vi "states FG.vi"(6 "exit in":bool, 8 "state # in":i32, 9 "subState in":T1, 10 "menu (get)":enum16{"set", "get"}(ring)=enum."get", 11 "Loop ID":i32) -> (0 "first call?":bool, 1 "exit out":bool, 2 "state # out":i32, 3 "subState out":T1=enum."driver control")   [LabVIEW 2013]
uses:
  typedefs/State Machine/subStates.ctl
panel:
  # "The All-Powerful Functional Global with all the States"
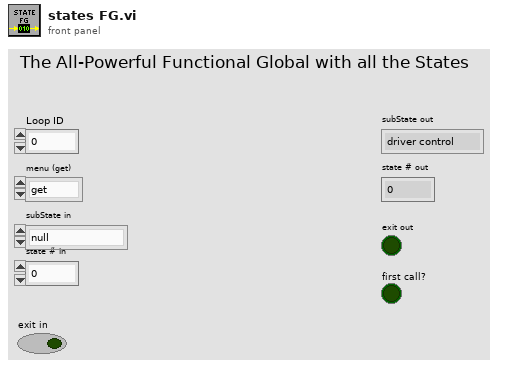
[diagram p1: front panel]
types:
  T1 = typedef "subStates.ctl" = enum16{"null", "wait", "driver control", "auto", "manual override", "hold position", "rotate", "pickup", "pass", "load", "goto shoot", "shoot high goal", "shoot low goal", "cancel arm", "cancel shooter", "end", "test"}
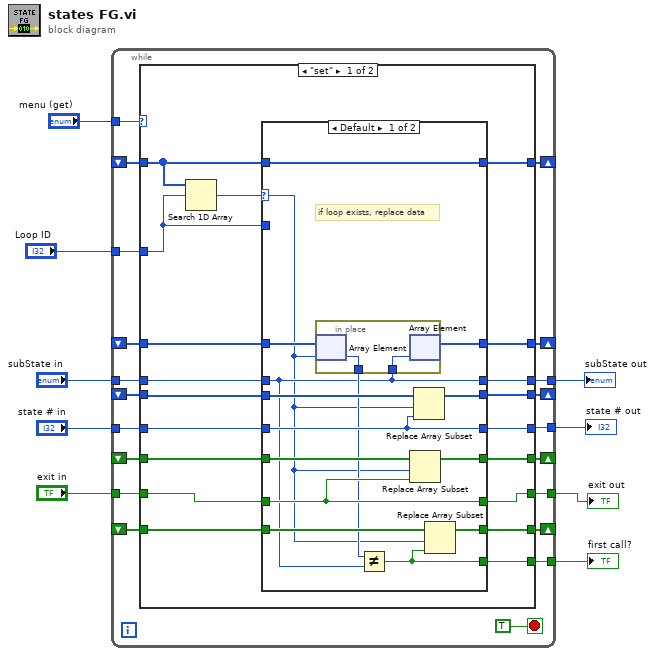
[diagram p0: block diagram]
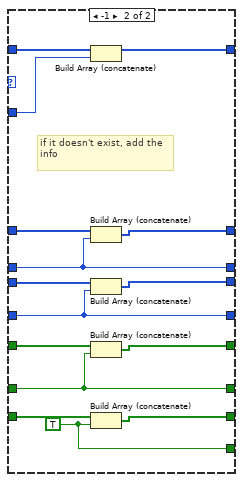
[diagram p2: hidden frame]
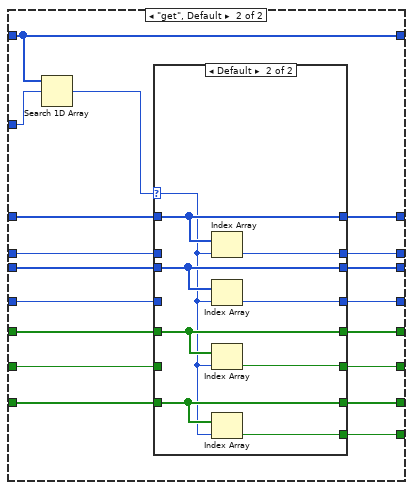
[diagram p3: hidden frame]
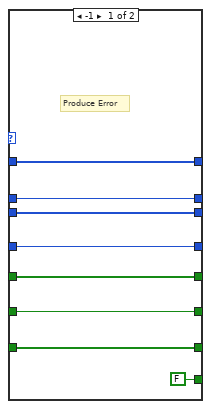
[diagram p4: hidden frame]
diagram:
  n1 = while {
    tunnel: "menu (get)" -> [w29]
    shift-right: [w24] -> _
    shift-left: _ -> [w25]
    shift-right: [w23] -> _
    shift-left: _ -> [w26]
    tunnel: "Loop ID" -> [w27]
    shift-right: [w21] -> _
    shift-left: _ -> [w22]
    tunnel: "subState in" -> [w20]
    tunnel: "state # in" -> [w19]
    tunnel: [w18] -> w5
    tunnel: [w17] -> w4
    shift-right: [w16] -> _
    shift-left: _ -> [w15]
    tunnel: [w14] -> w2
    tunnel: "exit in" -> [w13]
    shift-right: [w12] -> _
    shift-left: _ -> [w11]
    tunnel: [w10] -> w1
    stop <- TRUE stop-if-true
    n2 = case shown="\"set\"" w29 {
      tunnel: w27 -> [w46 w92]
      tunnel: w26 -> [w43 w98]
      tunnel: w25 -> [w45 w97]
      tunnel: [w40 w81] -> w18
      tunnel: [w41 w96] -> w24
      tunnel: [w39 w95] -> w23
      tunnel: [w38 w94] -> w17
      tunnel: w22 -> [w47 w91]
      tunnel: [w37 w91] -> w21
      tunnel: w20 -> [w44 w90]
      tunnel: w19 -> [w42 w89]
      tunnel: [w35 w88] -> w16
      tunnel: w15 -> [w36 w87]
      tunnel: [w34 w86] -> w14
      tunnel: w13 -> [w33 w85]
      tunnel: [w32 w83] -> w12
      tunnel: w11 -> [w31 w84]
      tunnel: [w30 w82] -> w10
      frame "set" {
        n3 = Search 1D Array(1D array=w47, element=w46) -> (index of element=w48:i32)  [unwired: 1 in]
        n4 = case shown="Default" w48 {
          selector: w48 -> [w49 _]
          tunnel: [w63 w80] -> w37
          tunnel: w47 -> [w63 w79]
          tunnel: w46 -> [_ w78]
          tunnel: w45 -> [w53 w77]
          tunnel: w44 -> [w50 w75]
          tunnel: [w52 w76] -> w41
          tunnel: [w50 w75] -> w40
          tunnel: w43 -> [w62 w74]
          tunnel: w42 -> [w60 w72]
          tunnel: [w61 w73] -> w39
          tunnel: [w60 w72] -> w38
          tunnel: w36 -> [w55 w71]
          tunnel: [w56 w70] -> w35
          tunnel: [w54 w69] -> w34
          tunnel: w33 -> [w54 w69]
          tunnel: [w59 w68] -> w32
          tunnel: w31 -> [w58 w67]
          tunnel: [w57 w66] -> w30
          frame Default {
            # "if loop exists, replace data"
            n5 = in-place {
              in-place-border: w50 -> [w65]
              in-place-border: [w64] -> w51
              n6 = in-place-array #1(w53, w49) -> (w64:T1)
              n7 = in-place-array #1(w65) -> (w52:T1[])  [unwired: 1 out]
            }
            n8 = Not Equal?(x=w51, y=w50) -> (x != y?=w57:bool)
            n9 = Replace Array Subset(array=w55, new element=w54, index=w49) -> (w56:bool[])
            n10 = Replace Array Subset(array=w62, new element=w60, index=w49) -> (w61:i32[])
            n11 = Replace Array Subset(array=w58, new element=w57, index=w49) -> (w59:bool[])
          }
          frame -1 {
            w66 = TRUE
            # "if it doesn't exist, add the info"
            n12 = Build Array (concatenate)(w79, w78) -> (w80:i32[])
            n13 = Build Array (concatenate)(w77, w75) -> (w76:T1[])
            n14 = Build Array (concatenate)(w74, w72) -> (w73:i32[])
            n15 = Build Array (concatenate)(w71, w69) -> (w70:bool[])
            n16 = Build Array (concatenate)(w67, w66) -> (w68:bool[])
          }
        }
      }
      frame "get", Default {
        n17 = Search 1D Array(1D array=w91, element=w92) -> (index of element=w93:i32)  [unwired: 1 in]
        n18 = case shown="Default" w93 {
          selector: w93 -> [_ w107]
          tunnel: w98 -> [w105 w113]
          tunnel: w97 -> [w106 w114]
          tunnel: [w104 w115] -> w81
          tunnel: [w106 w114] -> w96
          tunnel: [w105 w113] -> w95
          tunnel: [w103 w112] -> w94
          tunnel: w90 -> [w104 _]
          tunnel: w89 -> [w103 _]
          tunnel: [w102 w111] -> w88
          tunnel: w87 -> [w102 w111]
          tunnel: [w101 w110] -> w86
          tunnel: w85 -> [w101 _]
          tunnel: [w100 w109] -> w83
          tunnel: w84 -> [w100 w109]
          tunnel: [FALSE w108] -> w82
          frame -1 {
            # "Produce Error"
          }
          frame Default {
            n19 = Index Array(array=w114, index=w107) -> (element=w115:T1)
            n20 = Index Array(array=w113, index=w107) -> (element=w112:i32)
            n21 = Index Array(array=w111, index=w107) -> (element=w110:bool)
            n22 = Index Array(array=w109, index=w107) -> (element=w108:bool)
          }
        }
      }
    }
  }
  "subState out" <- w5
  "state # out" <- w4
  "exit out" <- w2
  "first call?" <- w1
